vi "Assignment W2.vi"() -> ()   [LabVIEW 2022 SP3]
panel:
  out "Average Grade":dbl format="%.2f"
  out "Grade 5":dbl
  out "Grade 4":dbl
  out "Grade 3":dbl
  out "Grade 2":dbl
  out "Grade 1":dbl
  out "Name 5":string
  out "Name 4":string
  out "Name 3":string
  out "Name 2":string
  out "Name 1":string
  in  "Stop continous loop update grades":bool
  out "Class Size":dbl
  in  "Class's Student input data":T1
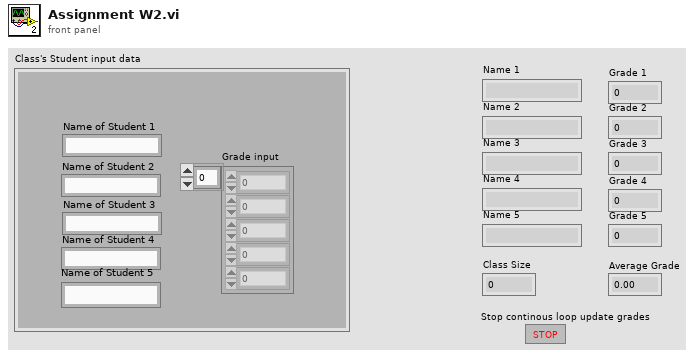
[diagram p1: front panel]
types:
  T1 = cluster{"Name of Student 1\n":string, "Name of Student 2\n":string, "Name of Student 3":string, "Name of Student 4\n":string, "Name of Student 5":string, "Grade input":dbl[]}
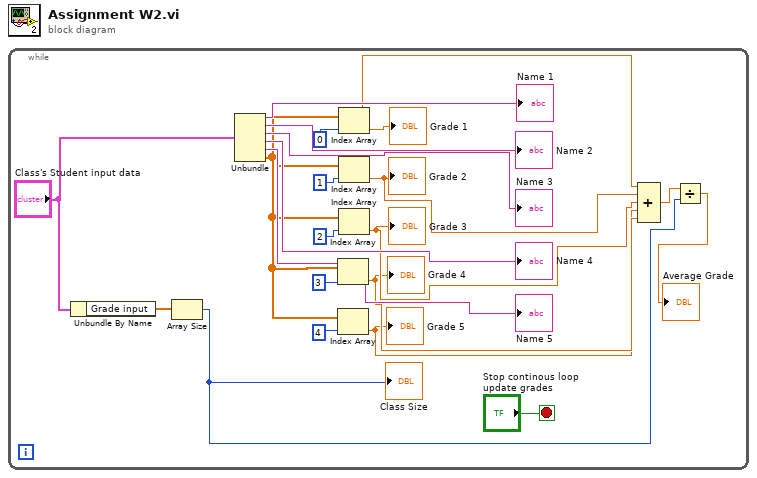
[diagram p0: block diagram]
diagram:
  n1 = while {
    stop <- "Stop continous loop update grades" stop-if-true
    n2 = Unbundle By Name("Class's Student input data") -> ("Grade input"=w2:dbl[])
    n3 = Array Size(array=w2) -> (size(s)=w1:i32)
    "Class Size" <- w1
    n4 = Unbundle("Class's Student input data") -> ("Name of Student 1"=→"Name 1":string, "Name of Student 2"=→"Name 2":string, "Name of Student 3"=→"Name 3":string, "Name of Student 4"=→"Name 4":string, "Name of Student 5"=→"Name 5":string, "Grade input"=w11:dbl[])
    n5 = Index Array(array=w11, index=3) -> (element=w7:dbl)
    "Grade 4" <- w7
    n6 = Index Array(array=w11, index=4) -> (element=w6:dbl)
    "Grade 5" <- w6
    n7 = Index Array(array=w11, index=0) -> (element=w10:dbl)
    "Grade 1" <- w10
    n8 = Index Array(array=w11, index=1) -> (element=w9:dbl)
    "Grade 2" <- w9
    n9 = Index Array(array=w11, index=2) -> (element=w8:dbl)
    "Grade 3" <- w8
    n10 = Compound Arithmetic op=ADD(w10, w9, w8, w6, w7) -> (w5:dbl)
    n11 = Divide(x=w5, y=w1) -> (x/y=→"Average Grade":dbl)
  }
